vi "Send Control Mouse Leave.vi"(9 "Time":u32, 10 "Ctl Refnum":refnum<vi>, 11 "Message Enqueuer in":refnum<class "Message Enqueuer.lvclass">) -> (0 "error out":errorcluster)   [LabVIEW 2018, in "MVA Framework.lvlib" / "ActorEvents.lvlib" / "ControlMouseLeaveMsg.lvclass"]
doc: "<License>\nCopyright © 2017 Composed Systems, LLC | All rights reserved\nwww.composed.io\n\nAuthor: Ethan Stern <ethan.stern@composed.io>\n\nThis software is provided \"AS IS\" WITHOUT WARRANTIES, either express or implied, AND IS FOR EDUCATIONAL PURPOSES ONLY.\n</License>"
uses:
  ControlMouseLeaveMsg.lvclass
  EventDataMessage/EventDataMessage.lvclass
  <vilib>/ActorFramework/Message Enqueuer/Message Enqueuer.lvclass
panel:
  in  "error in (no error)":errorcluster
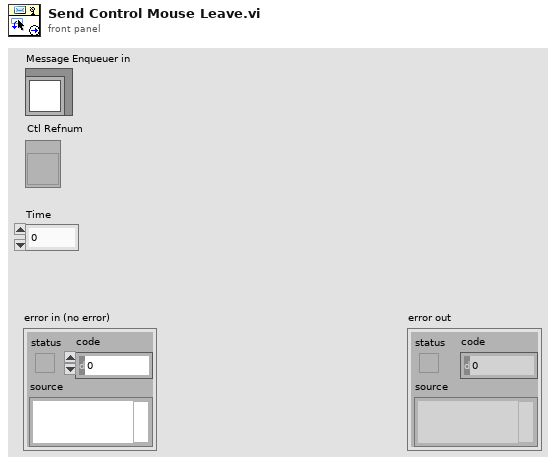
[diagram p1: front panel]
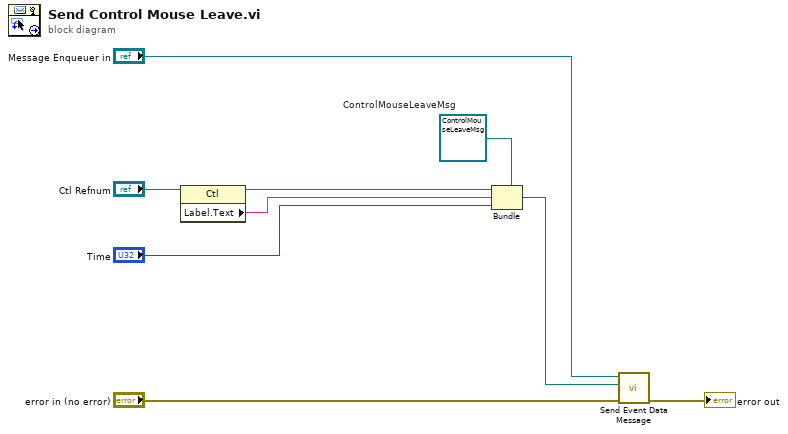
[diagram p0: block diagram]
diagram:
  w9 = refnum<class "ControlMouseLeaveMsg.lvclass"> refnum  # ControlMouseLeaveMsg
  n1 = property class="Ctl"(reference="Ctl Refnum") -> (reference out=w3:refnum<vi>, "Label.Text"=w2:string)  [unwired: 1 in, 1 out]
  n2 = Bundle(cluster=w9, w3, w2, "Time") -> (w6:refnum<class "ControlMouseLeaveMsg.lvclass">)
  n3 = call "Send Event Data Message.vi"("error in (no error)"="error in (no error)", "EventDataMessage"=w6, "Message Enqueuer in"="Message Enqueuer in") -> ("error out"=→"error out":errorcluster)  [unwired: 7 in, 1 out]
